vi "ReadHBMFileSARAHNewFile.vi"(4 "error in (no error)":errorcluster, 6 "file path":path) -> (0 "error out":errorcluster, 2 "HBMWaveformsOut":waveform(dbl)[](graph))   [LabVIEW 2017]
panel:
  out "TailleYAvant":i32[](array[numeric])
  out "dtAvant":dbl[](array[numeric])
  out "dtApres":dbl[](array[numeric])
  out "TailleYApres":i32[](array[numeric])
  out "size(s) 2":i32
  out "Waveform":waveform(dbl)[](graph)
  out "size(s)":i32
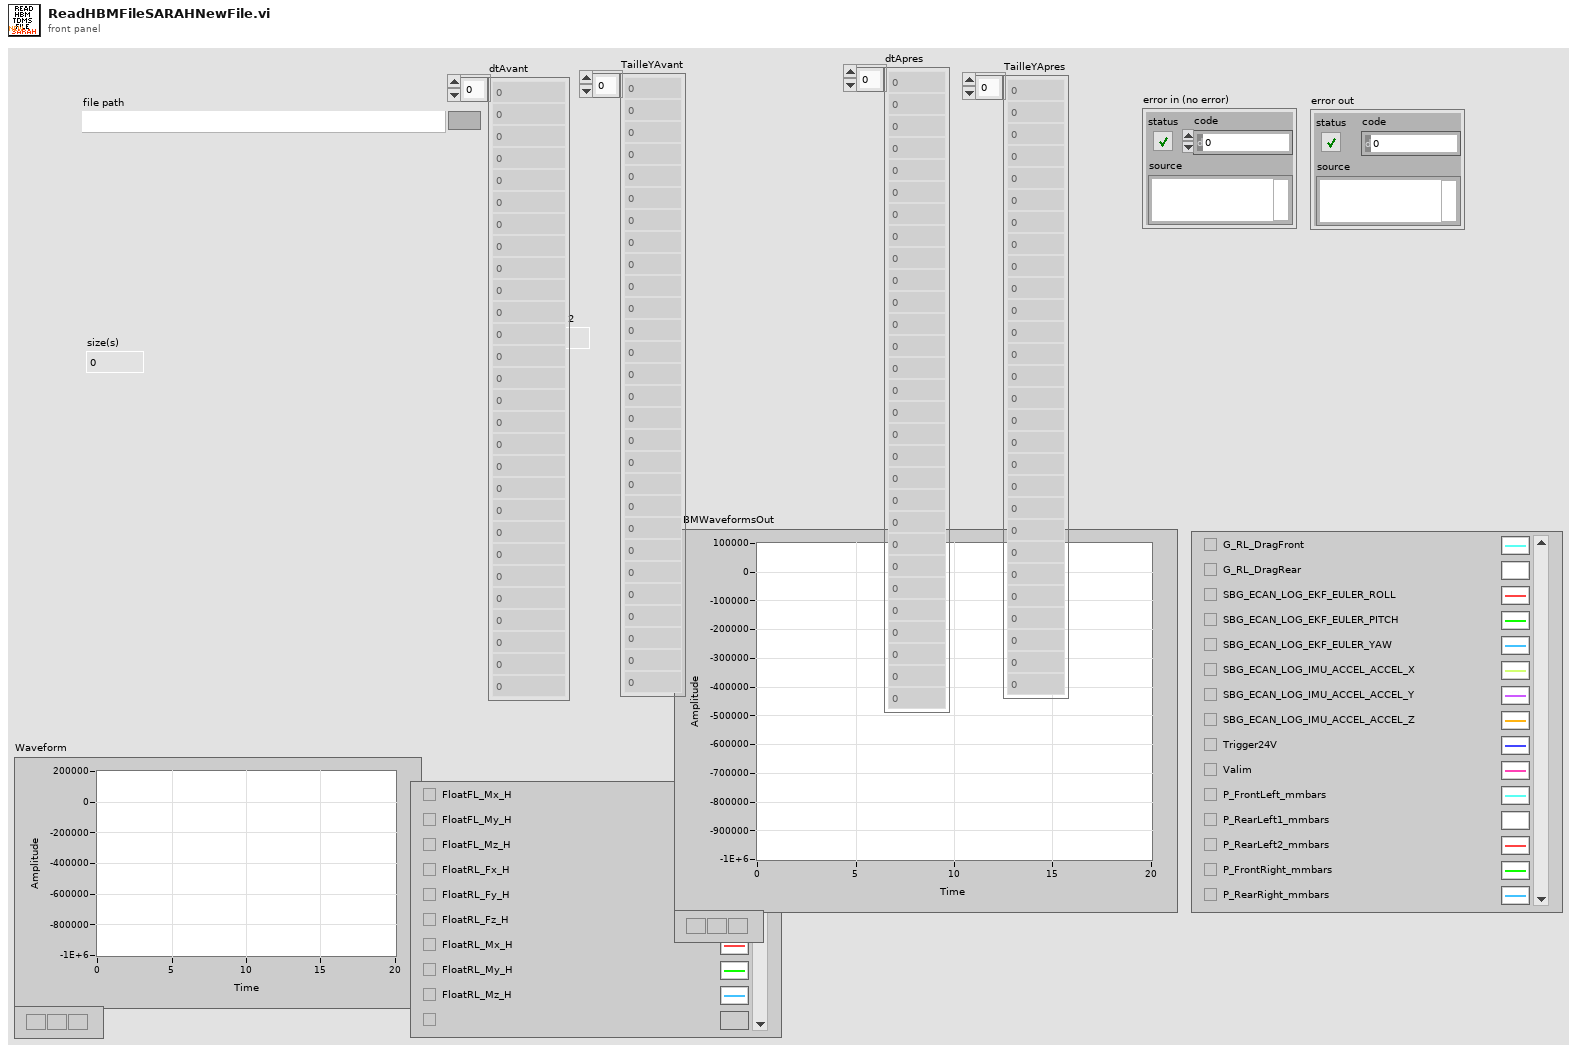
[diagram p1: front panel]
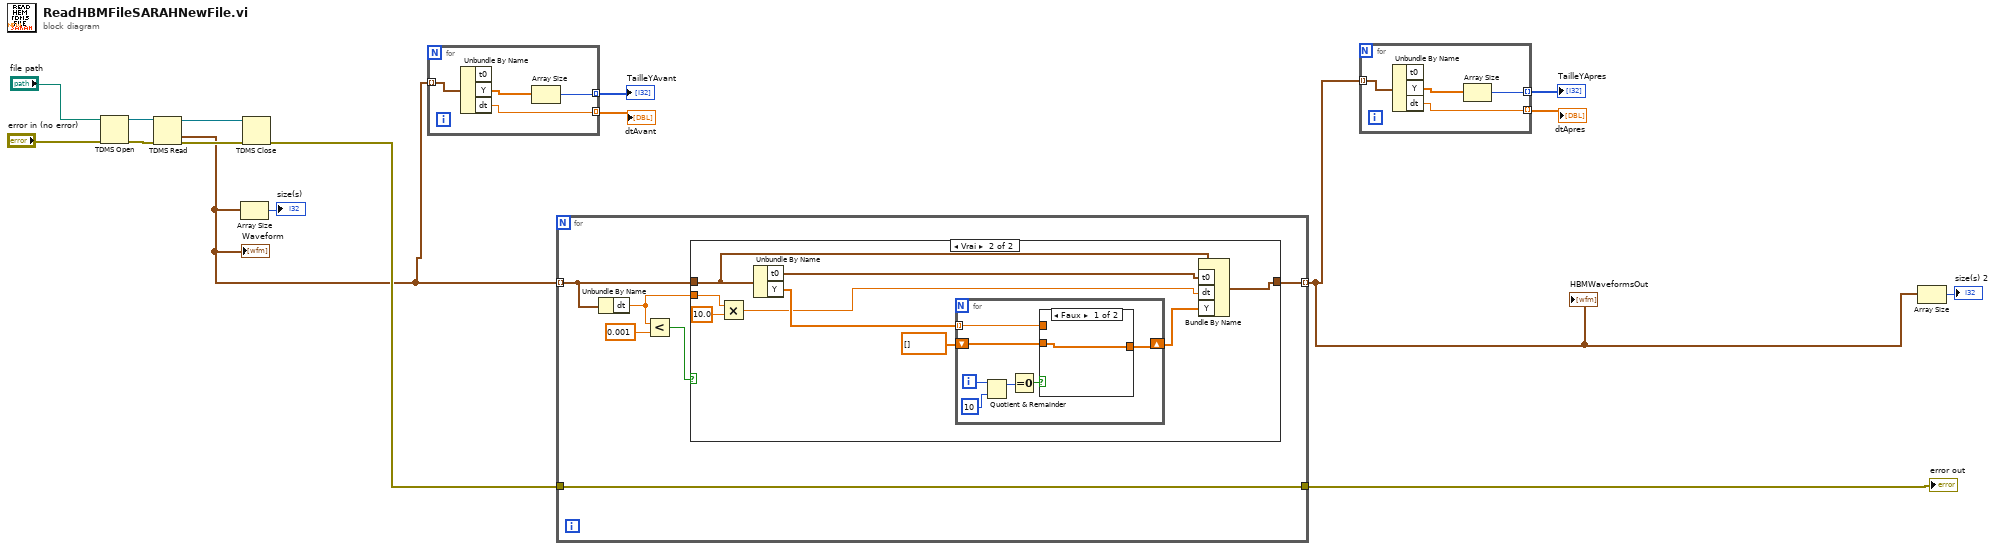
[diagram p0: block diagram]
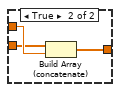
[diagram p3: hidden frame]
diagram:
  n1 = TDMS Open(8:"error in (no error)", 11:"file path") -> (0:w7:errorcluster, 3:w8:refnum<k34>)  [unwired: 5 in]
  n2 = TDMS Read(0:w8, 11:w7) -> (4:w5:refnum<k34>, 10:w3:waveform(dbl)[], 15:w6:errorcluster)  [unwired: 6 in, 3 out]
  "Waveform" <- w3
  n3 = Array Size(array=w3) -> (size(s)=→"size(s)":i32)
  n4 = TDMS Close(8:w6, 11:w5) -> (0:w4:errorcluster)  [unwired: 1 out]
  n5 = for {
    tunnel: w3 -> [w20] mode=indexing
    tunnel: [w18] -> w9 mode=indexing
    tunnel: [w17] -> w10 mode=indexing
    n6 = Unbundle By Name(w20) -> ("Y"=w19:dbl[], "dt"=w17:dbl)  [unwired: 1 out]
    n7 = Array Size(array=w19) -> (size(s)=w18:i32)
  }
  "TailleYAvant" <- w9
  "dtAvant" <- w10
  n8 = for {
    tunnel: w3 -> [w25] mode=indexing
    tunnel: [w24] -> w2 mode=indexing
    tunnel: w4 -> [w22]
    tunnel: [w22] -> w1
    n9 = Unbundle By Name(w25) -> ("dt"=w23:dbl)
    n10 = Less?(x=w23, y=0.001) -> (x < y?=w21:bool)
    n11 = case shown="Vrai" w21 {
      tunnel: w25 -> [w27 w28]
      tunnel: [w27 w29] -> w24
      tunnel: w23 -> [_ w35]
      frame False {
      }
      frame True {
        n12 = Multiply(x=w35, y=10.0) -> (x*y=w31:dbl)
        n13 = Unbundle By Name(w28) -> ("t0"=w32:timestamp, "Y"=w34:dbl[])
        n14 = for {
          tunnel: w34 -> [w40] mode=indexing
          shift-right: [w39] -> w30
          shift-left: dbl[] [] -> [w38]
          i -> [w43]
          n15 = Quotient & Remainder(x=w43, y=10) -> (x-y*floor(x/y)=w41:i32)  [unwired: 1 out]
          n16 = Equal To 0?(x=w41) -> (x = 0?=w37:bool)
          n17 = case shown="Faux" w37 {
            tunnel: w40 -> [_ w47]
            tunnel: [w44 w46] -> w39
            tunnel: w38 -> [w44 w45]
            frame False {
            }
            frame True {
              n18 = Build Array (concatenate)(w45, w47) -> (w46:dbl[])
            }
          }
        }
        n19 = Bundle By Name(cluster=w28, "t0"=w32, "dt"=w31, "Y"=w30) -> (w29:waveform(dbl))
      }
    }
  }
  "HBMWaveformsOut" <- w2
  "error out" <- w1
  n20 = for {
    tunnel: w2 -> [w51] mode=indexing
    tunnel: [w49] -> w12 mode=indexing
    tunnel: [w48] -> w11 mode=indexing
    n21 = Unbundle By Name(w51) -> ("Y"=w50:dbl[], "dt"=w48:dbl)  [unwired: 1 out]
    n22 = Array Size(array=w50) -> (size(s)=w49:i32)
  }
  "TailleYApres" <- w12
  "dtApres" <- w11
  n23 = Array Size(array=w2) -> (size(s)=→"size(s) 2":i32)
